vi "applicationControl.vi"() -> ()   [LabVIEW 2016]
panel:
  out "hasCanon":bool
  out "Saved?":bool
  in  "contstructingData":u8
  in  "totalScanFrame":dbl
  in  "currentScanFrame":dbl
  in  "scanAbort":bool
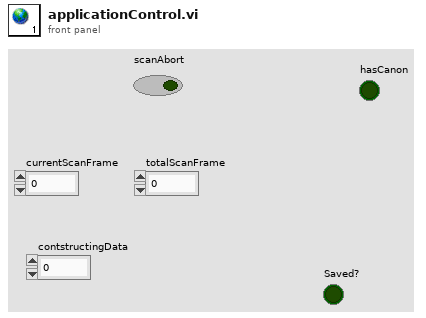
[diagram p1: front panel]
diagram:
